vi "Configure Level Trigger_20221208.vi"(0 "device session in":refnum<class "Device Session.lvclass">, 7 "Levels":T1={" Chan 0 trigger level hi (V)"=0.25, "Chan 0 trigger level lo (V) "=-0.25, " Chan 1 trigger level hi (V)"=0.25, "Chan 1 trigger level lo (V) "=-0.25, " Chan 2 trigger level hi (V)"=0.25, "Chan 2 trigger level lo (V) "=-0.25, " Chan 3 trigger level hi (V)"=0.25, "Chan 3 trigger level lo (V) "=-0.25, " Chan 4 trigger level hi (V)"=0.25, "Chan 4 trigger level lo (V) "=-0.25, " Chan 5 trigger level hi (V)"=0.25, "Chan 5 trigger level lo (V) "=-0.25, " Chan 6 trigger level hi (V)"=0.25, "Chan 6 trigger level lo (V) "=-0.25, " Chan 7 trigger level hi (V)"=0.25, "Chan 7 trigger level lo (V) "=-0.25}, 11 "error in":errorcluster) -> (4 "device session out":refnum<class "Device Session.lvclass">, 15 "error out":errorcluster)   [LabVIEW 2021, in "Device Session.lvclass"]
doc: "Configures the level trigger for a channel. You can specify the trigger slope, the trigger level, and whether the device should trigger on an input below or above the specified trigger level. You must run the <B>Configure Channel</B> VI before running this VI.\n\n<B>Input Parameters</B>\n\n<B>device session in</B> is a reference to the Device Session object, which contains a session to each instrument design library used in this sample project. This parameter is obtained from the 'Open Session' VI.\n\n<B>trigger source</B> specifies the channel to monitor for trigger conditions.\n\n<B>trigger when</B> specifies whether the device should trigger if the input is below or above the specified 'level'.\n\n<B>trigger level (V)</B> specifies the voltage threshold for the trigger.\n\n<B>instance</B> specifies either instance A or B of the trigger to use.\n\n<B>error in</B> describes error conditions that occur before this node runs. This input provides standard 'error in' functionality.\n\n<B>Output Parameters</B>\n\n<B>device session out</B> passes a reference to the session to the next VI.\n\n<B>error out</B> contains error information. This output provides standard 'error out' functionality."
uses:
  Device Session.lvclass
  Device Session.lvclass/Device Session.ctl
  <vilib>/Utility/error.llb/Error Cluster From Error Code.vi
  <vilib>/rvi/errors/niLvFpgaAdjustHostInterfaceError.vi
  <vilib>/rvi/interface/nirviReadWriteControl/nirviReadWriteControl.xnode
  FPGA Refnum.ctl
  NiFpgaLv.dll
  <vilib>/rvi/interface/Simulation/niFpgaSimulationCallBeginRW.vi
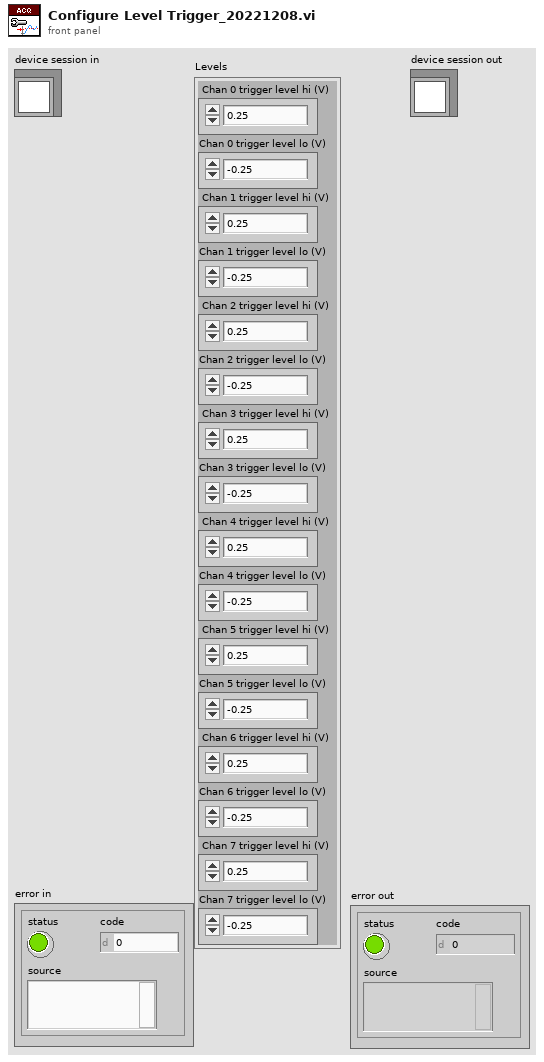
[diagram p1: front panel]
types:
  T1 = cluster{" Chan 0 trigger level hi (V)":dbl, "Chan 0 trigger level lo (V) ":dbl, " Chan 1 trigger level hi (V)":dbl, "Chan 1 trigger level lo (V) ":dbl, " Chan 2 trigger level hi (V)":dbl, "Chan 2 trigger level lo (V) ":dbl, " Chan 3 trigger level hi (V)":dbl, "Chan 3 trigger level lo (V) ":dbl, " Chan 4 trigger level hi (V)":dbl, "Chan 4 trigger level lo (V) ":dbl, " Chan 5 trigger level hi (V)":dbl, "Chan 5 trigger level lo (V) ":dbl, " Chan 6 trigger level hi (V)":dbl, "Chan 6 trigger level lo (V) ":dbl, " Chan 7 trigger level hi (V)":dbl, "Chan 7 trigger level lo (V) ":dbl}
  T2 = typedef "Device Session.lvclass/Device Session Object.ctl" = cluster{"fpga reference":T3, "reg bus":refnum<class "niInstr FIFO Register Bus v1 Host.lvclass">, "subsystem map":refnum<class "niInstr Subsystem Map v1 Host.lvclass">, "cal data":refnum<class "niHSAI Cal Data v1 Host.lvclass">, "config":refnum<class "niHSAI Group A Config v1 Host.lvclass">, "acquisition":refnum<class "niInstr Multirecord Acquisition v1 Host.lvclass">, "number of selected acq channels":u8, "selected acq channels":bool[], "number of channels":u32, "configured channels":bool[], "acq configuration":cluster{"number of samples":u64, "number of records":u64, "pretrigger samples":u64}, "actual channel configuration":T4[], "sample clock rate (Hz)":dbl, "scaling coefficients":T8[]}
  T3 = typedef "Device Session.lvclass/FPGA Refnum.ctl" = refnum<k20>
  T4 = typedef "niHSAI Types v1 Host.lvlib/Channel Configuration.ctl" = cluster{"channel":u32, "coupling":T5, "impedance":T6, "bandwidth":T7, "vertical range":dbl, "vertical offset":dbl}
  T5 = typedef "niHSAI Types v1 Host.lvlib/Coupling.ctl" = enum8{"Default", "DC", "AC"}
  T6 = typedef "niHSAI Types v1 Host.lvlib/Impedance.ctl" = enum8{"Default", "1 mega ohm", "50 ohm"}
  T7 = typedef "niHSAI Types v1 Host.lvlib/Bandwidth.ctl" = enum8{"Default", "Full Bandwidth", "Anti-alias Filter", "150 MHz"}
  T8 = typedef "niInstr Multirecord Acquisition v1 Host.lvclass/Scaling Coefficient.ctl" = cluster{"gain":dbl, "offset":dbl}
  T9 = typedef "niInstr Data Trigger v1 Shared.lvlib/Level Configuration FXP(+-,18,1).ctl" = cluster{"level":fxp<+/-,18,5>, "trigger when":T10}
  T10 = typedef "niInstr Data Trigger v1 Shared.lvlib/Level Configuration Trigger When.ctl" = enum8{"Trigger Above", "Trigger Below"}
  T11 = cluster{"configuration 2":T9, "configuration":T9}
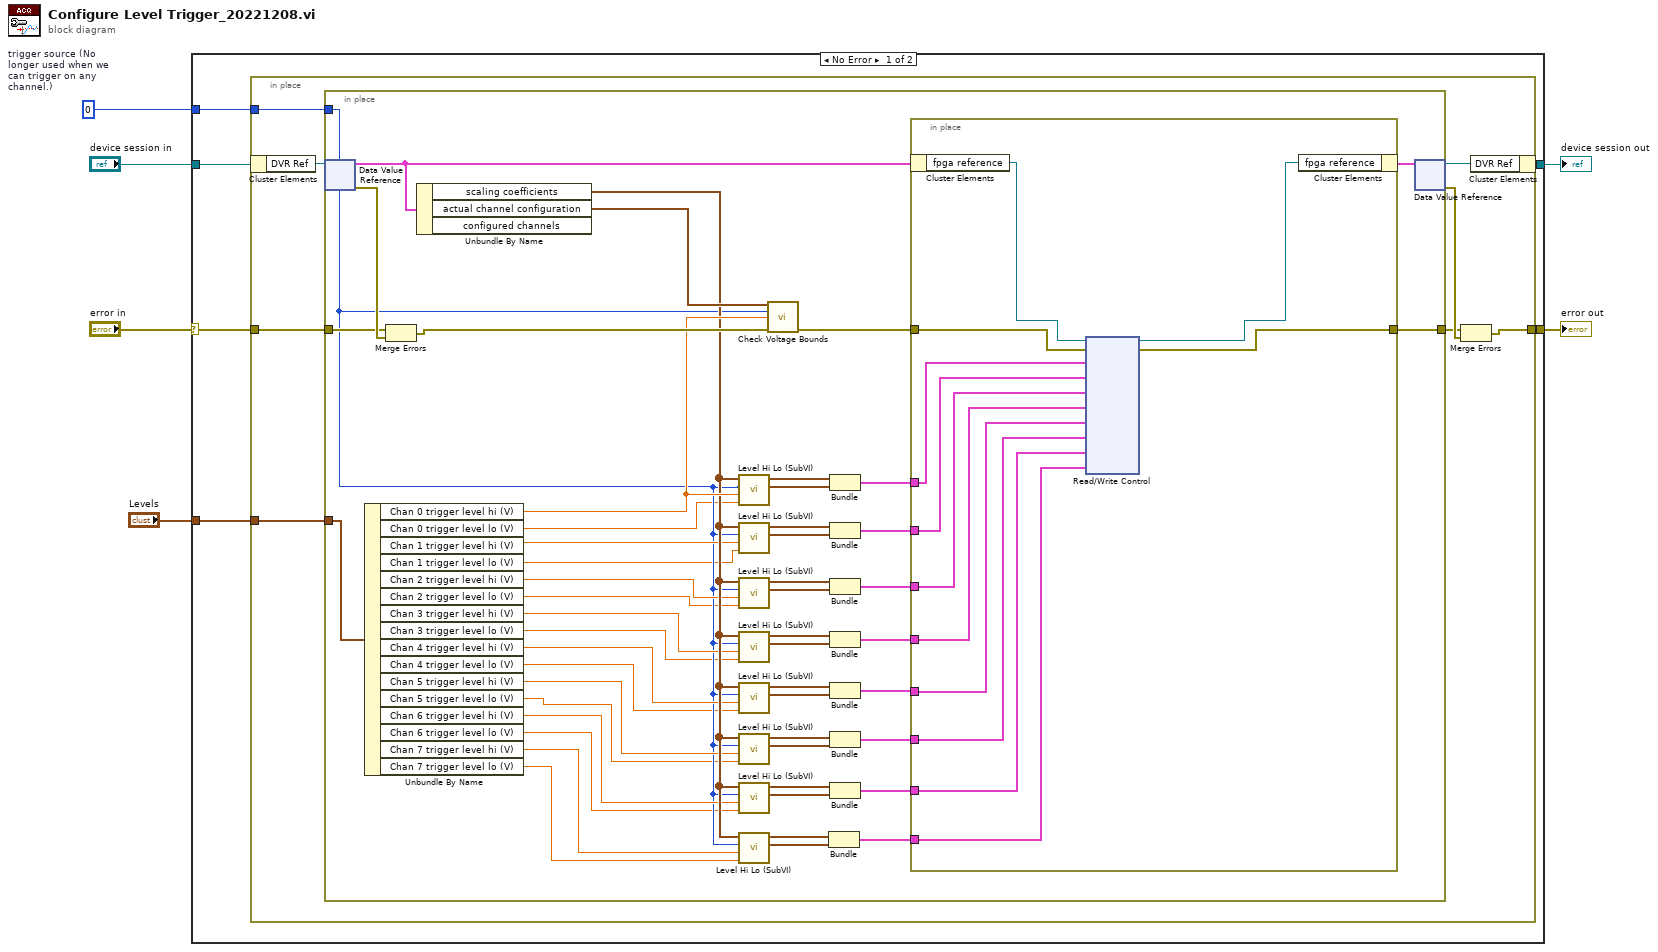
[diagram p0: block diagram]
diagram:
  w2 = u8 0  # trigger source (No longer used when we can trigger on any channel.)
  n1 = case shown="No Error" "error in" {
    selector: "error in" -> [w12 w85]
    tunnel: "device session in" -> [w9 w84]
    tunnel: [w8 w84] -> w5
    tunnel: [w10 w85] -> w6
    tunnel: w2 -> [w11 _]
    tunnel: "Levels" -> [w7 _]
    frame No Error {
      n2 = in-place {
        in-place-border: w12 -> [w20]
        in-place-border: w11 -> [w19]
        in-place-border: [w16] -> w10
        in-place-border: w7 -> [w13]
        n3 = in-place-cluster #1(w9) -> ("DVR Ref"=w15:refnum<data-value>)
        n4 = in-place {
          in-place-border: w20 -> [w70]
          in-place-border: w19 -> [w29]
          in-place-border: [w69] -> w17
          in-place-border: w13 -> [w63]
          n5 = in-place-dvr #2(w15) -> (w67:T2, w71:errorcluster)
          n6 = Unbundle By Name(w63) -> ("Chan 0 trigger level hi (V)"=w62:dbl, "Chan 0 trigger level lo (V)"=w28:dbl, "Chan 1 trigger level hi (V)"=w60:dbl, "Chan 1 trigger level lo (V)"=w27:dbl, "Chan 2 trigger level hi (V)"=w59:dbl, "Chan 2 trigger level lo (V)"=w26:dbl, "Chan 3 trigger level hi (V)"=w58:dbl, "Chan 3 trigger level lo (V)"=w25:dbl, "Chan 4 trigger level hi (V)"=w57:dbl, "Chan 4 trigger level lo (V)"=w24:dbl, "Chan 5 trigger level hi (V)"=w56:dbl, "Chan 5 trigger level lo (V)"=w23:dbl, "Chan 6 trigger level hi (V)"=w55:dbl, "Chan 6 trigger level lo (V)"=w22:dbl, "Chan 7 trigger level hi (V)"=w54:dbl, "Chan 7 trigger level lo (V)"=w21:dbl)
          n7 = Merge Errors(w70, w71) -> (w65:errorcluster)
          n8 = Unbundle By Name(w67) -> ("scaling coefficients"=w61:T8[], "actual channel configuration"=w64:T4[])  [unwired: 1 out]
          n9 = call "Level Hi Lo (SubVI).vi"("Chan 0 trigger level lo (V)"=w28, "Chan 0 trigger level hi (V)"=w62, "trigger source (No longer used when we can trigger on any channel.)"=w29, "scaling coefficients"=w61) -> ("configuration"=w52:T9, "configuration 2"=w53:T9)  [unwired: 6 in]
          n10 = call "Level Hi Lo (SubVI).vi"("Chan 0 trigger level lo (V)"=w27, "Chan 0 trigger level hi (V)"=w60, "trigger source (No longer used when we can trigger on any channel.)"=w29, "scaling coefficients"=w61) -> ("configuration"=w49:T9, "configuration 2"=w50:T9)  [unwired: 6 in]
          n11 = call "Level Hi Lo (SubVI).vi"("Chan 0 trigger level lo (V)"=w26, "Chan 0 trigger level hi (V)"=w59, "trigger source (No longer used when we can trigger on any channel.)"=w29, "scaling coefficients"=w61) -> ("configuration"=w46:T9, "configuration 2"=w47:T9)  [unwired: 6 in]
          n12 = call "Level Hi Lo (SubVI).vi"("Chan 0 trigger level lo (V)"=w25, "Chan 0 trigger level hi (V)"=w58, "trigger source (No longer used when we can trigger on any channel.)"=w29, "scaling coefficients"=w61) -> ("configuration"=w43:T9, "configuration 2"=w44:T9)  [unwired: 6 in]
          n13 = call "Level Hi Lo (SubVI).vi"("Chan 0 trigger level lo (V)"=w24, "Chan 0 trigger level hi (V)"=w57, "trigger source (No longer used when we can trigger on any channel.)"=w29, "scaling coefficients"=w61) -> ("configuration"=w41:T9, "configuration 2"=w42:T9)  [unwired: 6 in]
          n14 = call "Level Hi Lo (SubVI).vi"("Chan 0 trigger level lo (V)"=w23, "Chan 0 trigger level hi (V)"=w56, "trigger source (No longer used when we can trigger on any channel.)"=w29, "scaling coefficients"=w61) -> ("configuration"=w39:T9, "configuration 2"=w40:T9)  [unwired: 6 in]
          n15 = call "Level Hi Lo (SubVI).vi"("Chan 0 trigger level lo (V)"=w22, "Chan 0 trigger level hi (V)"=w55, "trigger source (No longer used when we can trigger on any channel.)"=w29, "scaling coefficients"=w61) -> ("configuration"=w37:T9, "configuration 2"=w38:T9)  [unwired: 6 in]
          n16 = call "Level Hi Lo (SubVI).vi"("Chan 0 trigger level lo (V)"=w21, "Chan 0 trigger level hi (V)"=w54, "trigger source (No longer used when we can trigger on any channel.)"=w29, "scaling coefficients"=w61) -> ("configuration"=w35:T9, "configuration 2"=w36:T9)  [unwired: 6 in]
          n17 = call "Check Voltage Bounds.vi"("channel configuration"=w64, "trigger source"=w29, "level (V)"=w62, "error in"=w65) -> ("error out"=w68:errorcluster)  [unwired: 11 in]
          n18 = Bundle("configuration 2"=w36, "configuration"=w35) -> (w30:T11)  [unwired: 1 in]
          n19 = Bundle("configuration 2"=w53, "configuration"=w52) -> (w51:T11)  [unwired: 1 in]
          n20 = Bundle("configuration 2"=w50, "configuration"=w49) -> (w48:T11)  [unwired: 1 in]
          n21 = Bundle("configuration 2"=w47, "configuration"=w46) -> (w45:T11)  [unwired: 1 in]
          n22 = Bundle("configuration 2"=w44, "configuration"=w43) -> (w34:T11)  [unwired: 1 in]
          n23 = Bundle("configuration 2"=w42, "configuration"=w41) -> (w33:T11)  [unwired: 1 in]
          n24 = Bundle("configuration 2"=w40, "configuration"=w39) -> (w32:T11)  [unwired: 1 in]
          n25 = Bundle("configuration 2"=w38, "configuration"=w37) -> (w31:T11)  [unwired: 1 in]
          n26 = in-place {
            in-place-border: [w83] -> w69
            in-place-border: w68 -> [w82]
            in-place-border: w51 -> [w79]
            in-place-border: w48 -> [w78]
            in-place-border: w45 -> [w77]
            in-place-border: w34 -> [w76]
            in-place-border: w33 -> [w75]
            in-place-border: w32 -> [w74]
            in-place-border: w31 -> [w73]
            in-place-border: w30 -> [w72]
            n27 = in-place-cluster #3(w67) -> ("fpga reference"=w80:T3)
            n28 = xnode "Read/Write Control"("FPGA VI Reference In"=w80, "error in"=w82, "trig 0"=w79, "trig 1"=w78, "trig 2"=w77, "trig 3"=w76, "trig 4"=w75, "trig 5"=w74, "trig 6"=w73, "trig 7"=w72) -> ("FPGA VI Reference Out"=w81:T3, "error out"=w83:errorcluster)
            n29 = in-place-cluster #3("fpga reference"=w81) -> (w66:T2)
          }
          n30 = in-place-dvr #2(w66) -> (w14:refnum<data-value>, w18:errorcluster)
        }
        n31 = Merge Errors(w17, w18) -> (w16:errorcluster)
        n32 = in-place-cluster #1("DVR Ref"=w14) -> (w8:refnum<class "Device Session.lvclass">)
      }
    }
    frame Error {
    }
  }
  "error out" <- w6
  "device session out" <- w5
